vi "Elevator Controller.vi"(8 "error in":errorcluster) -> ()   [LabVIEW 2018]
doc: "This VI executes continuously carrying out the current operation and responding to updates or new operations. It will often contain the timing or control code that is difficult to place directly in TeleOp. This VI generally opens all sensors and motors and isolates the rest of the robot code from knowing how the operations are carried out."
uses:
  <vilib>/Rock Robotics/WPI/Framework/Completion Status.ctl
  Elevator Setpoints.ctl
  Elevator Operations.ctl
  <vilib>/Rock Robotics/WPI/ThirdParty/Phoenix-LabVIEW/Motor Controller/Controls/CTRE_Phoenix_MotorControl_FeedbackDevice.ctl
  <vilib>/Rock Robotics/WPI/ThirdParty/Phoenix-LabVIEW/Motor Controller/Controls/CTRE_Phoenix_MotorControl_LimitSwitchNormal.ctl
  <vilib>/Rock Robotics/WPI/ThirdParty/Phoenix-LabVIEW/Motor Controller/Controls/CTRE_Phoenix_MotorControl_LimitSwitchSource_Local.ctl
  <vilib>/Rock Robotics/WPI/ThirdParty/Phoenix-LabVIEW/Motor Controller/Controls/CTRE_Phoenix_MotorControl_ControlMode.ctl
  <vilib>/Rock Robotics/WPI/ThirdParty/Phoenix-LabVIEW/Motor Controller/Get/CTRE_Phoenix_MotorController_GetSelectedSensorData.vi
  <vilib>/Rock Robotics/Network Tables/NT Write Number.vi
  Elevator Published Globals.vi
  <vilib>/Rock Robotics/WPI/ThirdParty/Phoenix-LabVIEW/Motor Controller/Get/CTRE_Phoenix_MotorController_GetLimitSwitchStates.vi
  <vilib>/Rock Robotics/Network Tables/NT Write Boolean.vi
  <vilib>/Rock Robotics/WPI/ThirdParty/Phoenix-LabVIEW/Motor Controller/Get/CTRE_Phoenix_MotorController_GetClosedLoopData.vi
panel:
  in  "Time LimitDebounce":u32=500
  in  "ElevatorStopRange":dbl=20.0 format="%#_13g"
  out "Waveform Chart":i32(graph)
  out "inches":dbl=8.0
  out "% error":i32(graph)
  out "Position (Raw Sensor Units)":i32=208
  out "Waveform Chart 2":T1(graph)
  in  "Acceleration":i32=75
  in  "Cruise Velocity":i32=70
  in  "F":dbl=10.0
  in  "P":dbl=13.0
  in  "I":dbl
  in  "D":dbl
  in  "Interactive Values":T2={"Operation"=enum."LiftForTime", "Setpoint"=0.5, "Duration"=1.0, "Button"=FALSE, "DistanceFromEnd"=0.0}
  out "Current\nCmd":string="Started at  12:26:25.181\nDefault: Reserve,  S 0.0, D 0.000000"
  in  "Buttons":cluster{"Execute Cmd":bool, "Abort Cmd":bool}
  out "Command Timing":cluster{"Start Time (ms)":u32, "Iterations":i32}={"Start Time (ms)"=346916, "Iterations"=0}
  out "Status":T4=enum."Incomplete"
  # "Tip: It may be helpful to observe inputs and sensor values.\nYou may also want to display tuning or debugging controls."
  # "Interactive Command: You may fill in the settings for a command\nand schedule it with the Execute button. You can observe and abort\nany command while fine tuning the code for the controller."
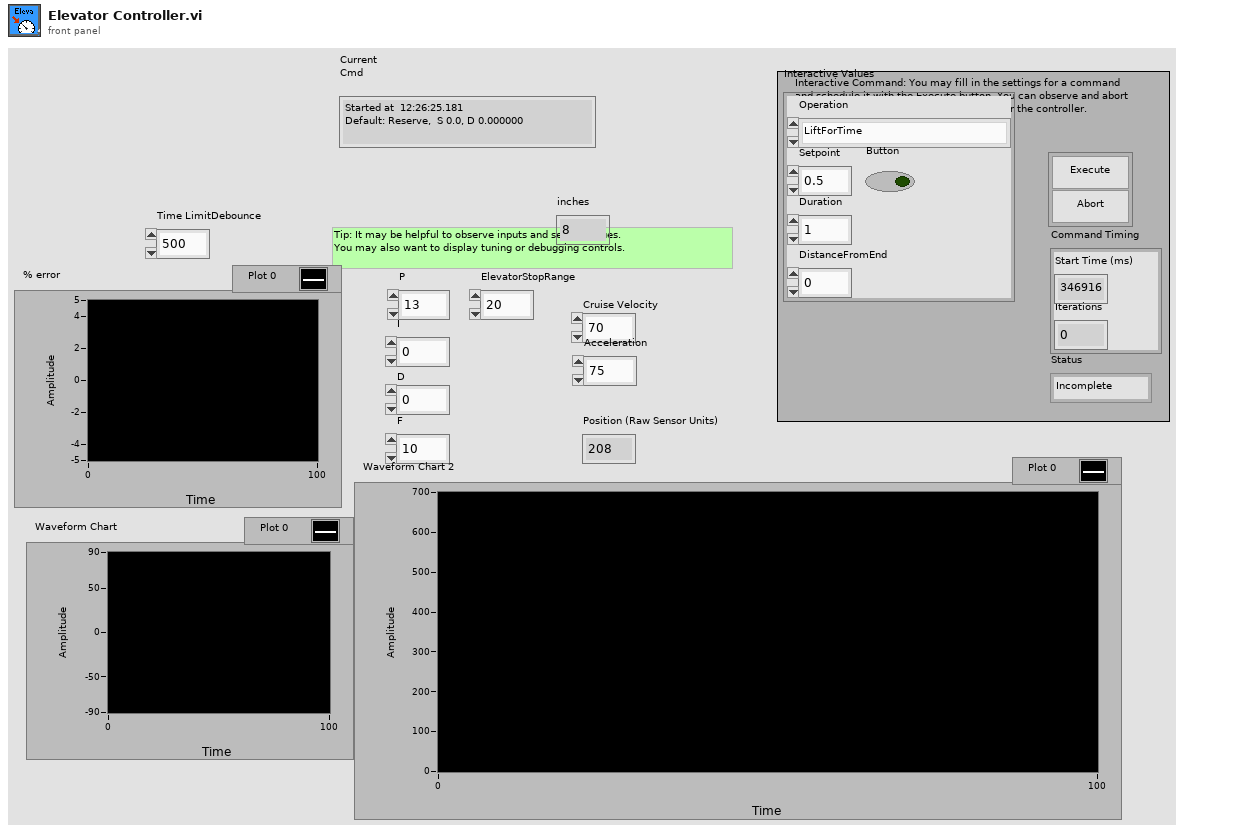
[diagram p1: front panel]
types:
  T1 = cluster{"Position (Raw Sensor Units)":i32, "Closed-loop Target":dbl}
  T2 = typedef "Elevator Setpoints.ctl" = cluster{"Operation":T3, "Setpoint":dbl, "Duration":dbl, "Button":bool, "DistanceFromEnd":dbl}
  T3 = typedef "Elevator Operations.ctl" = enum16{"Reserve", "Read Current", "Immediate", "GoToHeight", "StayAtHeight", "LiftForTime", "HeightAfterDriveAtDist"}
  T4 = typedef "Completion Status.ctl" = enum16{"Successful", "Aborted", "Incomplete"}
  T5 = typedef "CTRE_Phoenix_MotorControl_LimitSwitchSource_Local.ctl" = enum16{"Feedback Connector", "Remote Talon SRX", "Remote CANifier", "Deactivated"}
  T6 = typedef "CTRE_Phoenix_MotorControl_LimitSwitchNormal.ctl" = enum16{"Normally Open", "Normally Closed", "Disabled"}
  T7 = typedef "CTRE_Phoenix_MotorControl_FeedbackDevice.ctl" = i8
  T8 = typedef "WPI_MotorControlDeviceRef.ctl" = cluster{"DeviceStatus":errorcluster, "Type":T9, "PWM":cluster{"PWM Channel":T10, "DeadBand":T11}, "CAN":cluster{"Device Number":u8, "SetOutput VI Ref":variant, "GetOutput VI Ref":variant, "Enable VI Ref":variant, "Disable VI Ref":variant, "Data":variant}, "Invert":bool, "DIO PWM":cluster{"PWM \"Enable\" Channel":T10, "DIOChannel":T12, "PWM Rate":dbl}}
  T9 = typedef "WPI_MotorControlType.ctl" = enum16{"PWM", "CAN", "DIO PWM"}
  T10 = typedef "FPGA_DIOPWMChannel.ctl" = enum8{"PWM 0", "PWM 1", "PWM 2", "PWM 3", "PWM 4", "PWM 5", "PWM 6", "PWM 7", "PWM 8", "PWM 9", "PWM MXP 0", "PWM MXP 1", "PWM MXP 2", "PWM MXP 3", "PWM MXP 4", "PWM MXP 5", "PWM MXP 6", "PWM MXP 7", "PWM MXP 8", "PWM MXP 9", "Invalid"}
  T11 = typedef "WPI_PWMDeadband.ctl" = cluster{"Name":string, "maxPositivePwm":i32, "minPositivePwm":i32, "centerPwm":i32, "maxNegativePwm":i32, "minNegativePwm":i32, "angularRange":u16}
  T12 = typedef "FPGA_DIOChannel.ctl" = enum8{"DIO 0", "DIO 1", "DIO 2", "DIO 3", "DIO 4", "DIO 5", "DIO 6", "DIO 7", "DIO 8", "DIO 9", "DIO MXP 0", "DIO MXP 1", "DIO MXP 2", "DIO MXP 3", "DIO MXP 4", "DIO MXP 5", "DIO MXP 6", "DIO MXP 7", "DIO MXP 8", "DIO MXP 9", "DIO MXP 10", "DIO MXP 11", "DIO MXP 12", "DIO MXP 13", "DIO MXP 14", "DIO MXP 15", "SPI Port CS1", "SPI Port CS2", "SPI Port CS3", "SPI Port MISO", "SPI Port MOSI", "Invalid"}
  T13 = typedef "Command Status Info.ctl" = cluster{"Name":string, "Status":T4, "notifier out":T14}
  T14 = typedef "Completion Notifier.ctl" = refnum<notifier>
  T15 = cluster{"Current Command":T2, "Command Timing":cluster{"Start Time (ms)":u32, "Iterations":i32}, "Command Arguments":cluster{"Command Info":T13, "Description":string, "Default Command":T2, "queue out":refnum<queue>, "Subsystem Name":string}}
  T16 = typedef "CTRE_Phoenix_MotorControl_ControlMode.ctl" = u16
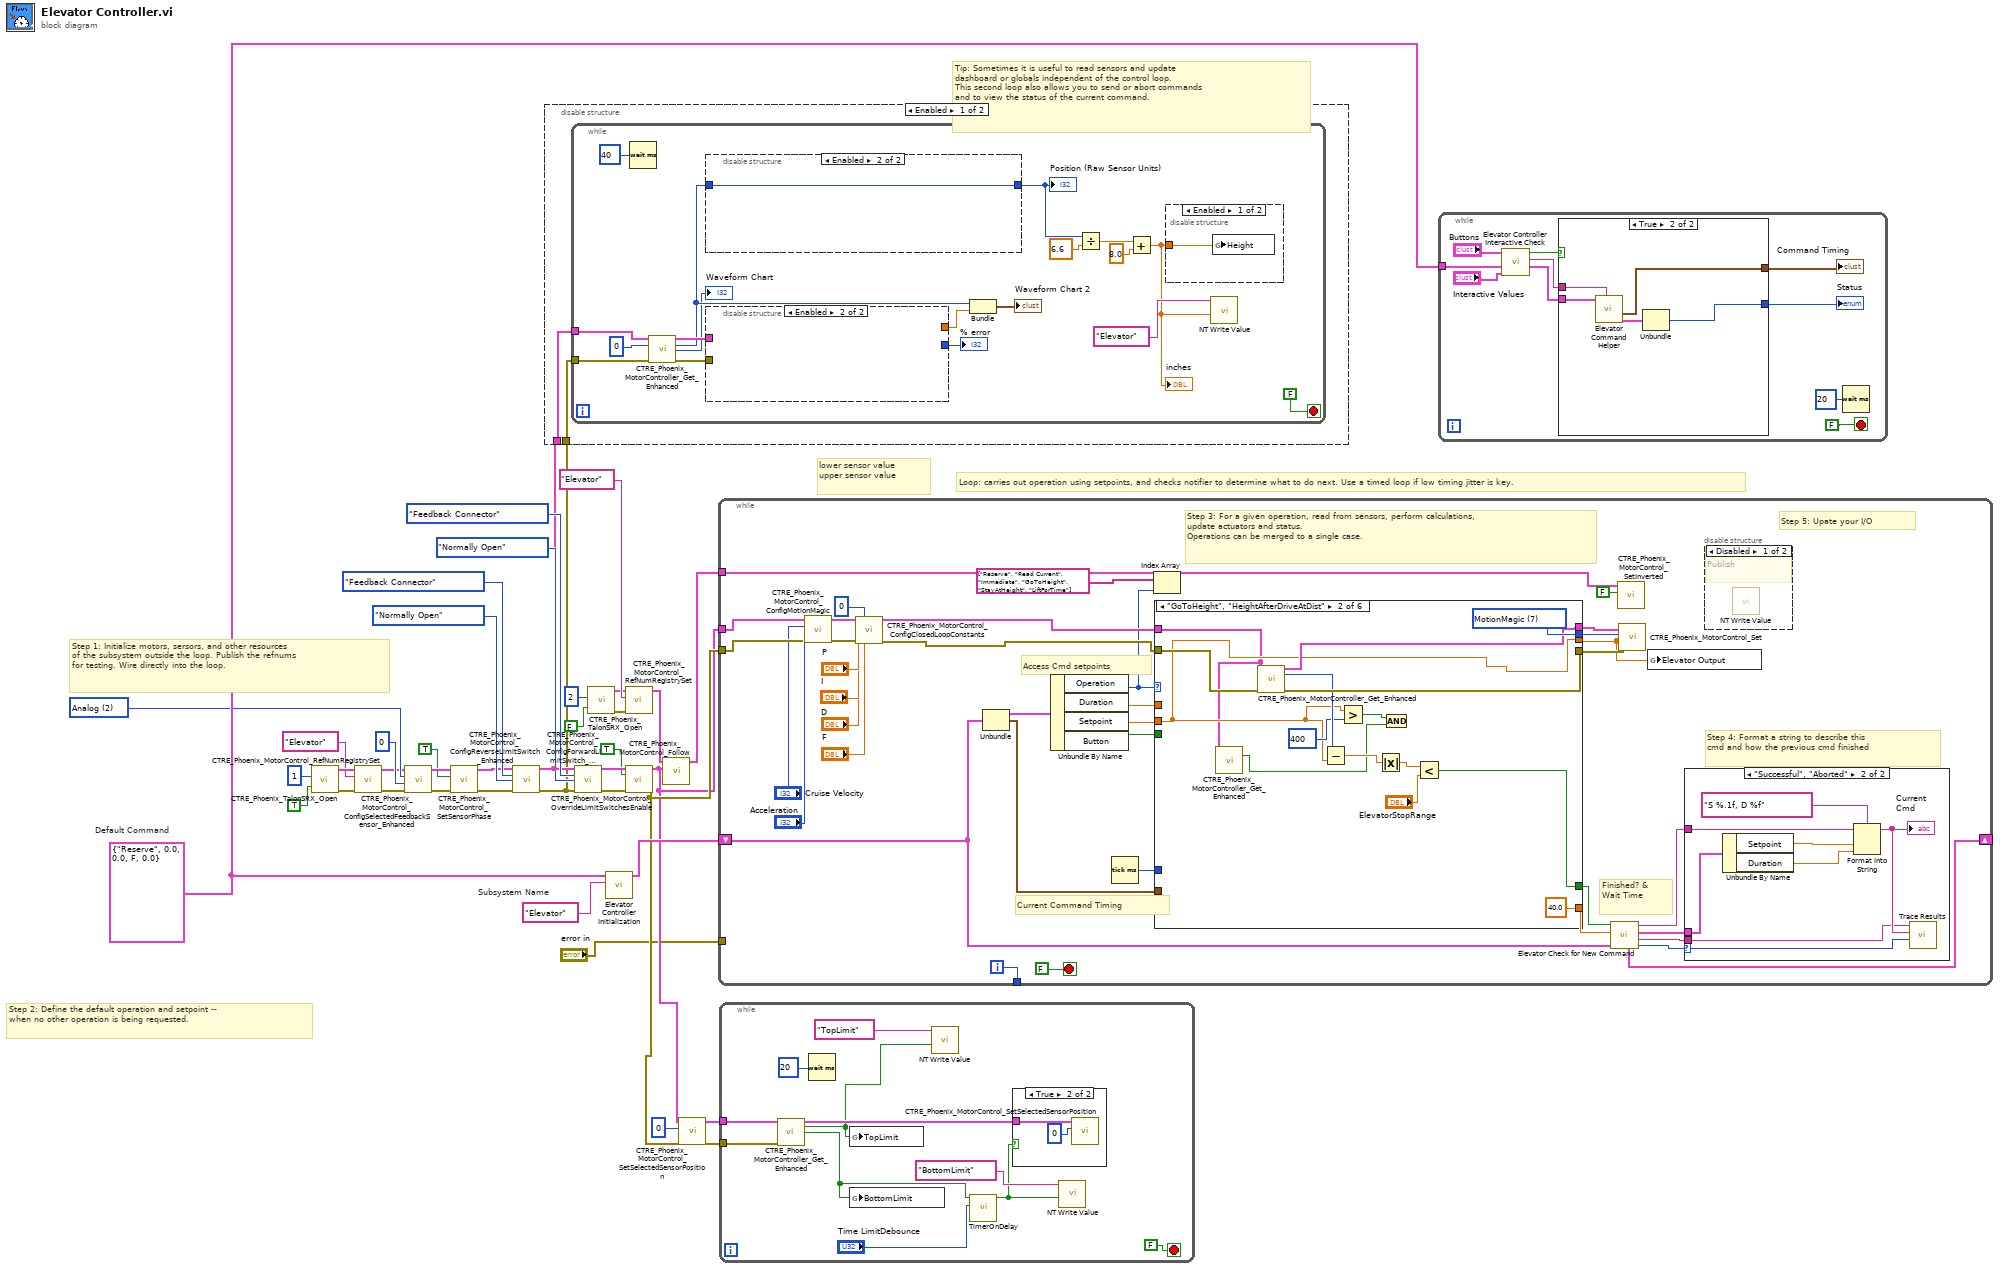
[diagram p0: block diagram]
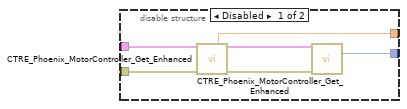
[diagram p3: hidden frame]
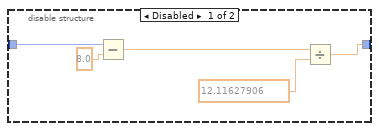
[diagram p5: hidden frame]
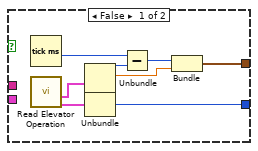
[diagram p7: hidden frame]
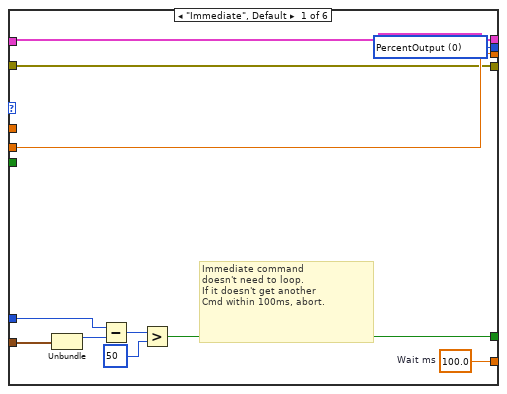
[diagram p10: hidden frame]
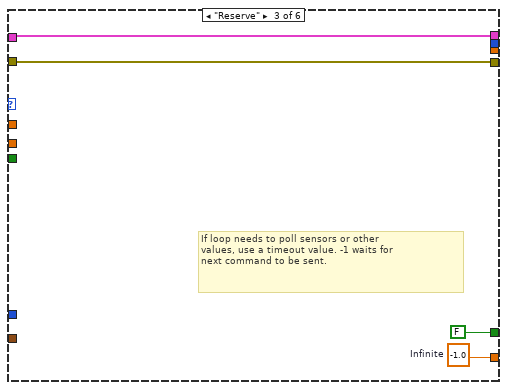
[diagram p11: hidden frame]
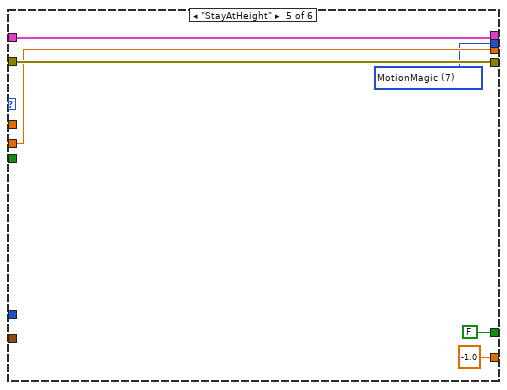
[diagram p13: hidden frame]
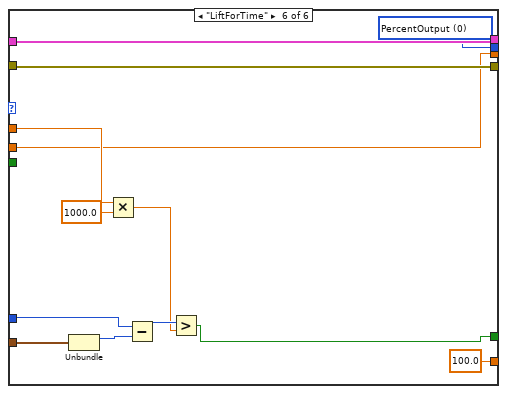
[diagram p14: hidden frame]
diagram:
  w30 = T7 2 items=["None"=-1, "QuadEncoder"=0, "Analog"=2, "Tachometer"=4, "Pulse Width Encoded Position"=8, "Sensor Sum (S0 + S1)"=9, "Sensor Difference (D0 - D1)"=10, "Remote Source 0"=11, "Remote Source 1"=12, "Software Emulated"=15] ("Feedback Device")
  w36 = T2 {"Operation"=enum."Reserve", "Setpoint"=0.0, "Duration"=0.0, "Button"=FALSE, "DistanceFromEnd"=0.0}  # Default Command
  w37 = "Elevator"  # Subsystem Name
  # "lower sensor value\nupper sensor value"
  # "Tip: Sometimes it is useful to read sensors and update\ndashboard or globals independent of the control loop.\nThis second loop also allows you to send or abort commands\nand to view the status of the current command."
  # "Step 2: Define the default operation and setpoint --\nwhen no other operation is being requested."
  # "Step 1: Initialize motors, sersors, and other resources\nof the subsystem outside the loop. Publish the refnums\nfor testing. Wire directly into the loop."
  # "Loop: carries out operation using setpoints, and checks notifier to determine what to do next. Use a timed loop if low timing jitter is key."
  n1 = call <vilib>:"CTRE_Phoenix_TalonSRX_Open.vi"("Invert"=TRUE, "Device Number"=u8 1) -> ("error out"=w34:errorcluster, "CAN Talon SRX Ref"=w35:T8)  [unwired: 8 in]
  n2 = call <vilib>:"CTRE_Phoenix_MotorControl_RefNumRegistrySet.vi"("error in (no error)"=w34, "refnum name"="Elevator", "PhoenixMotorControlDevRef"=w35) -> ("error out"=w31:errorcluster, "PhoenixMotorControlDevRef"=w13:T8)  [unwired: 7 in]
  n3 = call <vilib>:"CTRE_Phoenix_MotorControl_ConfigSelectedFeedbackSensor_Enhanced.vi"("error in (no error)"=w31, "pidLoopIdx"=0, "Feedback Device"=w30, "PhoenixMotorControlDevRef"=w13) -> ("error out"=w7:errorcluster, "PhoenixMotorControlDevRef"=w9:T8)  [unwired: 6 in]
  n4 = call <vilib>:"CTRE_Phoenix_MotorControl_SetSensorPhase.vi"("error in (no error)"=w7, "PhaseSensor"=TRUE, "PhoenixMotorControlDevRef"=w9) -> ("error out"=w6:errorcluster, "PhoenixMotorControlDevRef"=w8:T8)  [unwired: 7 in]
  n5 = call <vilib>:"CTRE_Phoenix_MotorControl_ConfigReverseLimitSwitch_Enhanced.vi"("PhoenixMotorControlDevRef"=w8, "Limit Switch Source"=CTRE_Phoenix_MotorControl_LimitSwitchSource_Local."Feedback Connector", "NormallyOpenOrClosed"=CTRE_Phoenix_MotorControl_LimitSwitchNormal."Normally Open", "error in (no error)"=w6) -> ("PhoenixMotorControlDevRef"=w21:T8, "error out"=w20:errorcluster)  [unwired: 10 in]
  n6 = disable-structure shown="Enabled" {
    disable-tunnel: w21 -> [w40 _]
    disable-tunnel: w20 -> [w39 _]
    frame Enabled {
      n7 = while {
        tunnel: w40 -> [w53]
        tunnel: w39 -> [w52]
        stop <- FALSE stop-if-true
        n8 = Wait (ms)(milliseconds to wait=u32 40) -> ()  [unwired: 1 out]
        n9 = call-poly <vilib>:"CTRE_Phoenix_MotorController_Get_Enhanced.vi"("PhoenixMotorControlDevRef"=w53, "pidLoopIdx"=u32 0, "error in"=w52) -> ("PhoenixMotorControlDevRef"=w57:T8, "Position (Raw Sensor Units)"=w48:i32, "Velocity (Raw Sensor Units per 100 ms)"=→"Waveform Chart":i32, "error out"=w51:errorcluster)  [unwired: 9 in]
        n10 = disable-structure shown="Enabled" {
          disable-tunnel: [w70 w71] -> w47
          disable-tunnel: w48 -> [w69 w71]
          frame Disabled {
            n11 = Subtract(x=w69, y=8.0) -> (x-y=w68:dbl)
            n12 = Divide(x=w68, y=12.11627906 ("x")) -> (x/y=w70:dbl)
          }
          frame Enabled {
          }
        }
        "Position (Raw Sensor Units)" <- w47
        n13 = disable-structure shown="Enabled" {
          disable-tunnel: w57 -> [w64 _]
          disable-tunnel: [w63 _] -> w56
          disable-tunnel: w51 -> [w62 _]
          disable-tunnel: [w59 _] -> w49
          frame Disabled {
            n14 = call-poly <vilib>:"CTRE_Phoenix_MotorController_Get_Enhanced.vi"("PhoenixMotorControlDevRef"=w64, "error in"=w62) -> ("Closed-loop Target"=w63:dbl, "PhoenixMotorControlDevRef"=w61:T8, "error out"=w60:errorcluster)  [unwired: 8 in, 3 out]
            n15 = call-poly <vilib>:"CTRE_Phoenix_MotorController_Get_Enhanced.vi"("PhoenixMotorControlDevRef"=w61, "error in"=w60) -> ("Closed-loop Error"=w59:i32)  [unwired: 8 in, 5 out]
          }
          frame Enabled {
          }
        }
        "% error" <- w49
        n16 = Bundle("Position (Raw Sensor Units)"=w48, "Closed-loop Target"=w56) -> (→"Waveform Chart 2":T1)  [unwired: 1 in]
        n17 = Divide(x=w47, y=6.6) -> (x/y=w44:dbl)
        n18 = Add(x=w44, y=8.0) -> (x+y=w41:dbl)
        "inches" <- w41
        n19 = disable-structure shown="Enabled" {
          disable-tunnel: w41 -> [w65 _]
          frame Enabled {
            n20 = global write "Elevator Published Globals.vi" "Height"(w65) -> ()
          }
          frame Disabled {
          }
        }
        n21 = call-poly <vilib>:"NT Write Value.vi"("Numeric"=w41, "Name"="Elevator") -> ()  [unwired: 9 in, 1 out]
      }
    }
    frame Disabled {
    }
  }
  n22 = call <vilib>:"CTRE_Phoenix_MotorControl_ConfigForwardLimitSwitch_Enhanced.vi"("PhoenixMotorControlDevRef"=w21, "Limit Switch Source"=CTRE_Phoenix_MotorControl_LimitSwitchSource_Local."Feedback Connector", "NormallyOpenOrClosed"=CTRE_Phoenix_MotorControl_LimitSwitchNormal."Normally Open", "error in (no error)"=w20) -> ("PhoenixMotorControlDevRef"=w24:T8, "error out"=w23:errorcluster)  [unwired: 10 in]
  n23 = call <vilib>:"CTRE_Phoenix_TalonSRX_Open.vi"("Invert"=FALSE, "Device Number"=u8 2) -> ("error out"=w17:errorcluster, "CAN Talon SRX Ref"=w16:T8)  [unwired: 8 in]
  n24 = call "Elevator Controller Initialization.vi"("Subsystem Name"=w37, "Default Command"=w36) -> ("Current Command"=w38:T15)  [unwired: 9 in]
  n25 = call <vilib>:"CTRE_Phoenix_MotorControl_RefNumRegistrySet.vi"("error in (no error)"=w17, "refnum name"="Elevator", "PhoenixMotorControlDevRef"=w16) -> ("PhoenixMotorControlDevRef"=w12:T8)  [unwired: 7 in, 1 out]
  n26 = call <vilib>:"CTRE_Phoenix_MotorControl_OverrideLimitSwitchesEnable.vi"("PhoenixMotorControlDevRef"=w24, "Override Limit Switch Enable?"=TRUE, "error in (no error)"=w23) -> ("PhoenixMotorControlDevRef"=w3:T8, "error out"=w10:errorcluster)  [unwired: 11 in]
  n27 = call <vilib>:"CTRE_Phoenix_MotorControl_Follow.vi"("Master Controller to Follow"=w3, "PhoenixMotorControlDevRef"=w12) -> ("PhoenixMotorControlDevRef"=w11:T8)  [unwired: 8 in, 1 out]
  n28 = call <vilib>:"CTRE_Phoenix_MotorControl_SetSelectedSensorPosition.vi"("New Sensor Position"=0, "PhoenixMotorControlDevRef"=w3) -> ("PhoenixMotorControlDevRef"=w2:T8)  [unwired: 8 in, 1 out]
  n29 = while {
    shift-right: [w102] -> _
    shift-left: w38 -> [w95]
    tunnel: [w107] -> _
    tunnel: "error in" -> [_]
    tunnel: w3 -> [w78]
    tunnel: w10 -> [w83]
    tunnel: w11 -> [w76]
    i -> [w107]
    stop <- FALSE stop-if-true
    # "Step 5: Upate your I/O"
    # "Step 4: Format a string to describe this\ncmd and how the previous cmd finished"
    # "Current Command Timing"
    # "Access Cmd setpoints"
    # "Finished? &\nWait Time"
    # "Step 3: For a given operation, read from sensors, perform calculations,\nupdate actuators and status.\nOperations can be merged to a single case."
    n30 = call <vilib>:"CTRE_Phoenix_MotorControl_ConfigMotionMagic.vi"("error in (no error)"=w83, "Acceleration"="Acceleration", "Cruise Velocity"="Cruise Velocity", "PhoenixMotorControlDevRef"=w78) -> ("error out"=w88:errorcluster, "PhoenixMotorControlDevRef"=w87:T8)  [unwired: 6 in]
    n31 = call <vilib>:"CTRE_Phoenix_MotorControl_ConfigClosedLoopConstants.vi"("PhoenixMotorControlDevRef"=w87, "slotIdx"=0, "P"="P", "I"="I", "D"="D", "error in (no error)"=w88, "F"="F") -> ("PhoenixMotorControlDevRef"=w80:T8, "error out"=w79:errorcluster)  [unwired: 7 in]
    n32 = Unbundle(w95) -> ("Current Command"=w106:T2, "Command Timing"=w104:cluster{"Start Time (ms)":u32, "Iterations":i32})  [unwired: 1 out]
    n33 = Unbundle By Name(w106) -> ("Operation"=w74:T3, "Duration"=w105:dbl, "Setpoint"=w103:dbl, "Button"=w82:bool)
    n34 = Tick Count (ms)() -> (millisecond timer value=w94:u32)
    n35 = Index Array(array=string[] ["Reserve", "Read Current", "Immediate", "GoToHeight", "StayAtHeight", "LiftForTime"] ("Strings []"), index=w74) -> ()  [unwired: 1 out]
    n36 = case shown="\"GoToHeight\", \"HeightAfterDriveAtDist\"" w74 {
      tunnel: [w127 40.0 ("Infinite") w146 _ -1.0 ("Infinite") 100.0 ("Infinite")] -> w100
      tunnel: [w121 w128 FALSE ("ignore previous (F)") _ FALSE ("ignore previous (F)") w160] -> w101
      tunnel: w104 -> [w123 _ _ _ _ w161]
      tunnel: w105 -> [_ _ _ _ _ w158]
      tunnel: w103 -> [w119 w132 _ _ w152 w155]
      tunnel: w80 -> [w117 w130 w144 w148 w154 w167]
      tunnel: w79 -> [w118 w140 w143 w147 w153 w166]
      tunnel: w94 -> [w122 _ _ _ _ w162]
      tunnel: [w118 w138 w143 w147 w153 w166] -> w93
      tunnel: [w117 w139 w144 w148 w154 w167] -> w92
      tunnel: [w119 w132 _ _ w152 w155] -> w72
      tunnel: [w120 w142 _ _ w150 w165] -> w75
      tunnel: w82 -> [_ _ _ _ _ _]
      frame "Immediate", Default {
        w120 = T16 0 items=["PercentOutput"=0, "Position"=1, "Velocity"=2, "Current"=3, "Follower"=5, "MotionProfile"=6, "MotionMagic"=7, "MotionMagicArc"=8, "MotionProfileArc"=10, "Disabled"=15] ("Control Mode")
        w127 = 100.0  # Wait ms
        # "Immediate command\ndoesn't need to loop.\nIf it doesn't get another\nCmd within 100ms, abort."
        n37 = Unbundle(w123) -> ("Start Time (ms)"=w126:u32)  [unwired: 1 out]
        n38 = Subtract(x=w122, y=w126) -> (x-y=w125:u32)
        n39 = Greater?(x=w125, y=u8 50 ("Left Motor")) -> (0:w121:bool)
      }
      frame "GoToHeight", "HeightAfterDriveAtDist" {
        w142 = T16 7 items=["PercentOutput"=0, "Position"=1, "Velocity"=2, "Current"=3, "Follower"=5, "MotionProfile"=6, "MotionMagic"=7, "MotionMagicArc"=8, "MotionProfileArc"=10, "Disabled"=15] ("Control Mode")
        n40 = call-poly <vilib>:"CTRE_Phoenix_MotorController_Get_Enhanced.vi"("PhoenixMotorControlDevRef"=w130) -> ("Forward Limit Closed?"=w129:bool)  [unwired: 11 in, 3 out]
        n41 = call-poly <vilib>:"CTRE_Phoenix_MotorController_Get_Enhanced.vi"("PhoenixMotorControlDevRef"=w130, "error in"=w140) -> ("PhoenixMotorControlDevRef"=w139:T8, "Position (Raw Sensor Units)"=w134:i32, "error out"=w138:errorcluster)  [unwired: 10 in, 1 out]
        n42 = Subtract(x=w134, y=w132) -> (x-y=w137:dbl)
        n43 = Greater?(x=w132, y=400) -> (0:w131:bool)
        n44 = Absolute Value(x=w137) -> (abs(x)=w136:dbl)
        n45 = And(x=w131, y=w129) -> ()  [unwired: 1 out]
        n46 = Less?(x=w136, y="ElevatorStopRange") -> (x < y?=w128:bool)
      }
      frame "Reserve" {
        w146 = -1.0  # Infinite
        # "If loop needs to poll sensors or other\nvalues, use a timeout value. -1 waits for\nnext command to be sent."
      }
      frame "Read Current" {
      }
      frame "StayAtHeight" {
        w150 = T16 7 items=["PercentOutput"=0, "Position"=1, "Velocity"=2, "Current"=3, "Follower"=5, "MotionProfile"=6, "MotionMagic"=7, "MotionMagicArc"=8, "MotionProfileArc"=10, "Disabled"=15] ("Control Mode")
      }
      frame "LiftForTime" {
        w165 = T16 0 items=["PercentOutput"=0, "Position"=1, "Velocity"=2, "Current"=3, "Follower"=5, "MotionProfile"=6, "MotionMagic"=7, "MotionMagicArc"=8, "MotionProfileArc"=10, "Disabled"=15] ("Control Mode")
        n47 = Unbundle(w161) -> ("Start Time (ms)"=w163:u32)  [unwired: 1 out]
        n48 = Multiply(x=w158, y=1000.0) -> (x*y=w157:dbl)
        n49 = Subtract(x=w162, y=w163) -> (x-y=w164:u32)
        n50 = Greater?(x=w164, y=w157) -> (0:w160:bool)
      }
    }
    n51 = call "Elevator Check for New Command.vi"("Current Command"=w95, "Wait time (ms)"=w100, "Finished?"=w101) -> ("Completion"=w96:T4, "Subsystem Name"=w97:string, "Current Command"=w98:T2, "Initial Trace String"=w99:string, "NextCommand"=w102:T15)  [unwired: 4 in]
    n52 = call <vilib>:"CTRE_Phoenix_MotorControl_SetInverted.vi"("Invert?"=FALSE, "PhoenixMotorControlDevRef"=w76) -> ()  [unwired: 8 in, 2 out]
    n53 = call <vilib>:"CTRE_Phoenix_MotorControl_Set.vi"("error in (no error)"=w93, "Output"=w72, "Control Mode"=w75, "PhoenixMotorControlDevRef"=w92) -> ()  [unwired: 6 in, 2 out]
    n54 = global write "Elevator Published Globals.vi" "Elevator Output"(w72) -> ()
    n55 = case shown="\"Successful\", \"Aborted\"" w96 {
      selector: w96 -> [_ w116]
      tunnel: w99 -> [_ w112]
      tunnel: w98 -> [_ w113]
      tunnel: w97 -> [_ w109]
      frame "Incomplete", Default {
        # "Continuing current command"
      }
      frame "Successful", "Aborted" {
        # "Report and setup for next command"
        n56 = Unbundle By Name(w113) -> ("Setpoint"=w115:dbl, "Duration"=w110:dbl)
        n57 = Format Into String(format string="S %.1f, D %f", initial string=w112, w115, w110) -> (resulting string=w111:string)  [unwired: 1 in, 1 out]
        "Current\nCmd" <- w111
        n58 = call <vilib>:"Trace Results.vi"("Status of previous command"=w116, "Description"=w111, "Subsystem"=w109) -> ()  [unwired: 9 in]
      }
    }
    n59 = disable-structure shown="Disabled" {
      frame Disabled {
        # "Publish"
        n60 = call-poly <vilib>:"NT Write Value.vi"() -> ()  [unwired: 11 in, 1 out]
      }
      frame Enabled {
      }
    }
  }
  n61 = while {
    tunnel: w2 -> [w177]
    tunnel: w10 -> [w178]
    stop <- FALSE stop-if-true
    n62 = call-poly <vilib>:"CTRE_Phoenix_MotorController_Get_Enhanced.vi"("PhoenixMotorControlDevRef"=w177, "error in"=w178) -> ("PhoenixMotorControlDevRef"=w175:T8, "Forward Limit Closed?"=w168:bool, "Reverse Limit Closed?"=w169:bool)  [unwired: 10 in, 1 out]
    n63 = Wait (ms)(milliseconds to wait=u32 20 ("millisecond timer value")) -> ()  [unwired: 1 out]
    n64 = global write "Elevator Published Globals.vi" "TopLimit"(w168) -> ()
    n65 = global write "Elevator Published Globals.vi" "BottomLimit"(w169) -> ()
    n66 = call-poly <vilib>:"NT Write Value.vi"("Boolean"=w168, "Name"="TopLimit") -> ()  [unwired: 9 in, 1 out]
    n67 = call "TimerOnDelay.vi"("Time Limit"="Time LimitDebounce", "Input"=w169) -> ("Output"=w171:bool)  [unwired: 9 in]
    n68 = case shown="True" w171 {
      tunnel: w175 -> [_ w180]
      frame False {
      }
      frame True {
        n69 = call <vilib>:"CTRE_Phoenix_MotorControl_SetSelectedSensorPosition.vi"("New Sensor Position"=0, "PhoenixMotorControlDevRef"=w180) -> ()  [unwired: 8 in, 2 out]
      }
    }
    n70 = call-poly <vilib>:"NT Write Value.vi"("Boolean"=w171, "Name"="BottomLimit") -> ()  [unwired: 9 in, 1 out]
  }
  n71 = while {
    tunnel: w36 -> [w187]
    stop <- FALSE stop-if-true
    n72 = call "Elevator Controller Interactive Check.vi"("Interactive Command in"="Interactive Values", "Default Command"=w187, "Buttons"="Buttons") -> ("Interactive Command out"=w184:T2, "Trace String"=w185:string, "Schedule"=w186:bool)  [unwired: 6 in]
    n73 = case shown="True" w186 {
      tunnel: [w198 w203] -> w183
      tunnel: w184 -> [_ w201]
      tunnel: [w194 w199] -> w182
      tunnel: w185 -> [_ w202]
      frame False {
        n74 = Tick Count (ms)() -> (millisecond timer value=w193:u32)
        n75 = call "Read Elevator Operation.vi"() -> ("Command Info"=w191:T13, "SubSystem Data"=w192:T2)  [unwired: 9 in, 1 out]
        n76 = Unbundle(w192) -> ("Operation"=w197:T3, "Setpoint"=w195:dbl)  [unwired: 3 out]
        n77 = Unbundle(w191) -> ("Status"=w198:T4)  [unwired: 2 out]
        n78 = Subtract(x=w193, y=w197) -> (x-y=w196:u32)
        n79 = Bundle(w196, "Setpoint"=w195) -> (w194:cluster{u32, "Setpoint":dbl})  [unwired: 1 in]
      }
      frame True {
        n80 = call "Elevator Command Helper.vi"("Description"=w202, "SubSystem Data"=w201) -> ("Command Info Out"=w200:T13, "Command Timing"=w199:cluster{"Start Time (ms)":u32, "Iterations":i32})  [unwired: 7 in, 1 out]
        n81 = Unbundle(w200) -> ("Status"=w203:T4)  [unwired: 2 out]
      }
    }
    "Status" <- w183
    "Command Timing" <- w182
    n82 = Wait (ms)(milliseconds to wait=u32 20) -> ()  [unwired: 1 out]
  }
